vi "User DLL.vi"(0 "Button 1":bool, 5 "Button 2":bool, 11 "Error in":errorcluster) -> (15 "Error out":errorcluster)   [LabVIEW 2020, in "LV Connectivity.lvlib"]
doc: "This VI used to look out for the implementation of user event from built in dlls of the windows files and this is used to auto click different buttons alternatively in specific interval."
uses:
  LV Connectivity.lvlib
  User32.dll
panel:
  # "USER32 DLL IMPLEMENTATION"
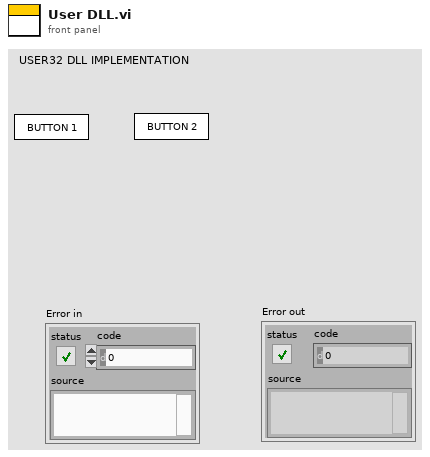
[diagram p1: front panel]
types:
  T1 = typedef "LVRectTypeDef.ctl" = cluster{"Left":i16, "Top":i16, "Right":i16, "Bottom":i16}
  T2 = typedef "LVPositionTypeDef.ctl" = cluster{"Left":i32, "Top":i32}
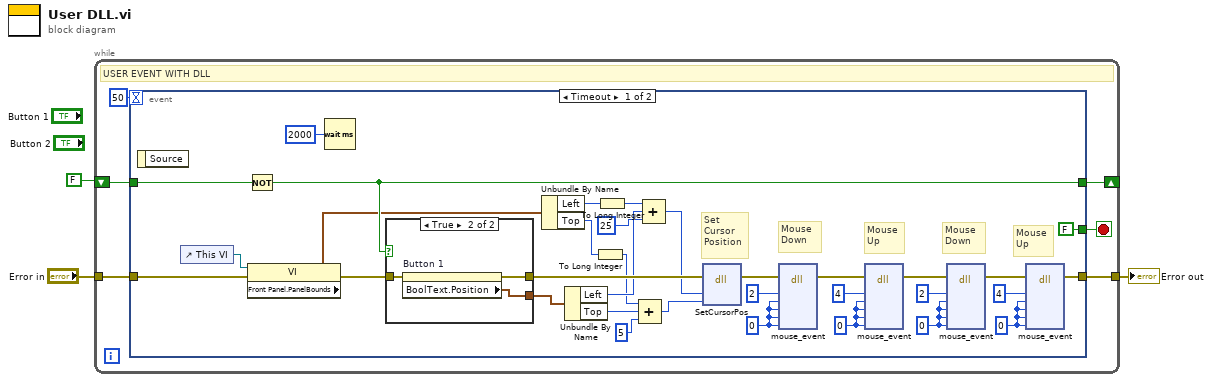
[diagram p0: block diagram]
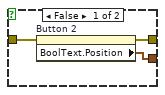
[diagram p2: hidden frame]
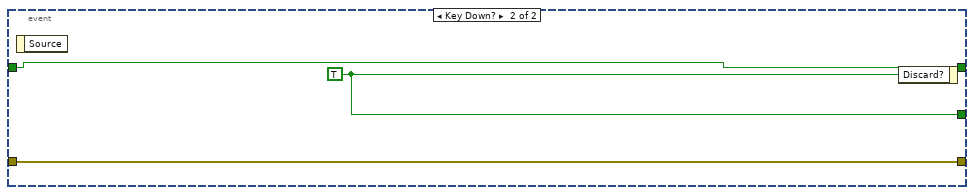
[diagram p3: hidden frame]
diagram:
  n1 = while {
    tunnel: "Error in" -> [w8]
    tunnel: [w7] -> w2
    shift-right: [w4] -> _
    shift-left: FALSE -> [w5]
    stop <- w9 stop-if-true
    # "USER EVENT WITH DLL"
    n2 = event shown="[0] Timeout" {
      selector: _ -> [_ _]
      dyn-events: _ -> [_ _]
      timeout: 50 -> [_ _]
      tunnel: [FALSE ("Discard?") w51] -> w9
      tunnel: w8 -> [w41 w50]
      tunnel: [w25 w50] -> w7
      tunnel: w5 -> [w39 w49]
      tunnel: [w37 w49] -> w4
      event Timeout {
        w30 = 0 ("In1")
        w32 = 0 ("In1")
        w33 = 0 ("In1")
        w35 = 0 ("In1")
        # "Set\nCursor\nPosition"
        # "Mouse\nUp"
        # "Mouse \nDown"
        # "Mouse\nUp"
        # "Mouse \nDown"
        n3 = event-data() -> ()  [unwired: 1 in, 1 out]
        n4 = control-ref of="This VI"() -> (w40:refnum<vi>)
        n5 = Not(x=w39) -> (.not. x?=w37:bool)
        n6 = property class="VI"(reference=w40, error in=w41) -> (error out=w38:errorcluster, "Front Panel.PanelBounds"=w20:T1)  [unwired: 1 out]
        n7 = Wait (ms)(milliseconds to wait=u32 2000) -> ()  [unwired: 1 out]
        n8 = case shown="True" w37 {
          tunnel: w38 -> [w45 w48]
          tunnel: [w44 w47] -> w24
          tunnel: [w43 w46] -> w22
          frame False {
            n9 = property on="Button 2" class="Bool"(error in=w45) -> (error out=w44:errorcluster, "BoolText.Position"=w43:T2)  [unwired: 1 in, 1 out]
          }
          frame True {
            n10 = property on="Button 1" class="Bool"(error in=w48) -> (error out=w47:errorcluster, "BoolText.Position"=w46:T2)  [unwired: 1 in, 1 out]
          }
        }
        n11 = Unbundle By Name(w20) -> ("Left"=w18:i16, "Top"=w17:i16)
        n12 = Unbundle By Name(w22) -> ("Left"=w19:i32, "Top"=w13:i32)
        n13 = To Long Integer(number=w17) -> (32bit integer=w14:i32)
        n14 = To Long Integer(number=w18) -> (32bit integer=w16:i32)
        n15 = Compound Arithmetic op=ADD(w14, w13, 5 ("value")) -> (w10:i32)
        n16 = Compound Arithmetic op=ADD(w16, w19, 25 ("value")) -> (w11:i32)
        n17 = dll-call lib="User32.dll" fn="SetCursorPos"(error in=w24, "arg1"=w11, "arg2"=w10) -> (error out=w23:errorcluster)  [unwired: 5 in, 1 out]
        n18 = dll-call lib="User32.dll" fn="mouse_event"(error in=w23, "In5"=2, "In2"=w35, "In3"=w35, "In4"=w35, "In1"=w35) -> (error out=w28:errorcluster)  [unwired: 8 in, 1 out]
        n19 = dll-call lib="User32.dll" fn="mouse_event"(error in=w28, "In5"=4, "In2"=w33, "In3"=w33, "In4"=w33, "In1"=w33) -> (error out=w27:errorcluster)  [unwired: 8 in, 1 out]
        n20 = dll-call lib="User32.dll" fn="mouse_event"(error in=w27, "In5"=2, "In2"=w30, "In3"=w30, "In4"=w30, "In1"=w30) -> (error out=w26:errorcluster)  [unwired: 8 in, 1 out]
        n21 = dll-call lib="User32.dll" fn="mouse_event"(error in=w26, "In5"=4, "In2"=w32, "In3"=w32, "In4"=w32, "In1"=w32) -> (error out=w25:errorcluster)  [unwired: 8 in, 1 out]
      }
      event Key Down? {
        w51 = TRUE ("Discard?")
        n22 = event-data() -> ()  [unwired: 1 in, 1 out]
        n23 = event-data("Discard?"=w51) -> ()  [unwired: 1 in, 1 out]
      }
    }
  }
  "Error out" <- w2
